vi "TEST-JSON-RPC.vi"() -> ()   [LabVIEW 2019]
uses:
  TEST-JSON-RPC--Cluster.ctl
  <vilib>/JDP Science/JSONtext/JSON Value Type.ctl
  JSON-RPC/JSON-RPC.lvclass/JSON-RPC.ctl
  <vilib>/numeric/Random Number (Range) DBL.vi
  1676b8f3-5053-426b-a1fc-41622b99c0bd.vi
  91eee69d-f7a9-4e42-a9d1-dd5bf5c27f07.vi
  9d079c85-1838-48ae-a1c4-15f57872b121.vi
  423c0946-e876-4033-917c-c4e0f5a656b4.vi
  0ae8443b-0c4b-4e01-b233-50273e00e751.vi
  6f47a901-0ffd-4612-bb45-9ae4cf78a1c3.vi
  f8f63b4b-b52f-497a-b775-281fe5a76cc4.vi
  9d79f0c2-35ce-467d-8164-7d449b6aa026.vi
  53d3177d-6787-4563-b3f2-ec7d47ca270a.vi
  d9266a12-4538-4804-ad7c-12d0542650b7.vi
  JSON-RPC/private/Write ids.vi
  JSON-RPC/private/Read ids.vi
  JSON-RPC/private/Parse Response-JSONtext.vi
  <vilib>/JDP Science/JSONtext/JSON text to Variant (path).vi
  JSON-RPC/private/Parse Response-JSONtext.vi/7ce7fba8-9f44-478d-b6cb-b571ff29f2f5.vi
  JSON-RPC/private/Parse Response-JSONtext.vi/8c905beb-ab4c-49e3-b5c6-2c663b7b30d7.vi
  JSON-RPC/private/Parse Response-JSONtext.vi/fce5892e-0c40-47e1-88e0-6c122aadefe2.vi
  <vilib>/JDP Science/JSONtext/Find Item.vi
  <vilib>/JDP Science/JSONtext/String Subset.vi
  JSON-RPC/private/Create Request-JSONtext.vi
  <vilib>/JDP Science/JSONtext/support/Format JSON Array Text.vi
  <vilib>/JDP Science/JSONtext/JSON text to Variant.vi
  JSON-RPC/private/Create Response-JSONtext.vi
  <vilib>/JDP Science/JSONtext/Get Array Elements.vi
  <vilib>/JDP Science/JSONtext/Get all Object Items.vi
  <vilib>/JDP Science/JSONtext/Parsing/Parse Full Path or Item Name.vi
  <vilib>/JDP Science/JSONtext/Next JSON Value.vi
  <vilib>/JDP Science/JSONtext/support/Error Cluster From Code.vi
  <vilib>/JDP Science/JSONtext/Offset/Find Item Locations by Path.vi
  <vilib>/Utility/error.llb/Error Cluster From Error Code.vi
  <vilib>/Utility/Data Type/Get Type Information.vi
  JSON-RPC/JSON-RPC.lvclass
  <vilib>/JDP Science/JSONtext/LVClass Serializer/JSONtext LVClass Serializer.lvclass
  <vilib>/JDP Science/JSONtext/JSONtext.lvlib
  <vilib>/numeric/Random Number (Range) I64.vi
panel:
  out "Array":T1[](array[typedef])
  out "Names 3":string[](array[string])
  out "Params 3":string[](array[string])
  out "Clusters Section":dbl[](array[numeric])
  out "Arrays":dbl[][](array[numeric])
  out "Clusters":T2[](array[typedef])
  out "Params 2":string[](array[string])
  out "Names 2":string[](array[string])
  out "Params":string[](array[string])
  out "Names":string[](array[string])
  out "REQ.Methods":string[](array[string])
  out "Match?":bool[](array[boolean])
  out "{JSON} Response":string
  out "{JSON} Requests":string
  out "4. parse response":dbl format="%#_6p"
  out "3. create response":dbl format="%#_6p"
  out "2. parse request":dbl format="%#_6p"
  out "1. create request":dbl format="%#_6p"
  out "REQ.Params":string[](array[string])
  out "results":string[](array[string])
  in  "Numeric":i32=3
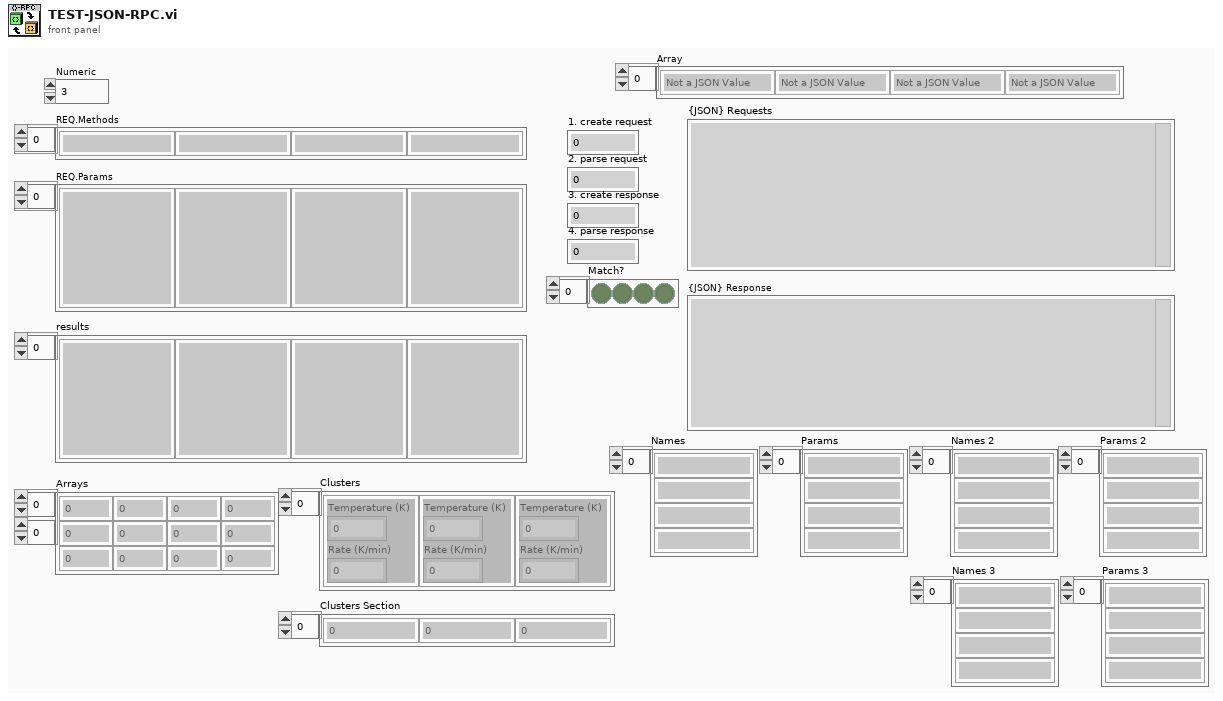
[diagram p1: front panel]
types:
  T1 = typedef "JSONtext.lvlib/JSON Value Type.ctl" = enum16{"Not a JSON Value", "JSON Object", "JSON Array", "String", "Number", "true", "false", "null"}
  T2 = typedef "TEST-JSON-RPC--Cluster.ctl" = cluster{"Temperature (K)":dbl, "Rate (K/min)":dbl}
  T3 = enum16{"Parse Error", "Invalid Request", "Method not found", "Invalid params", "Internal error", "Server error"}
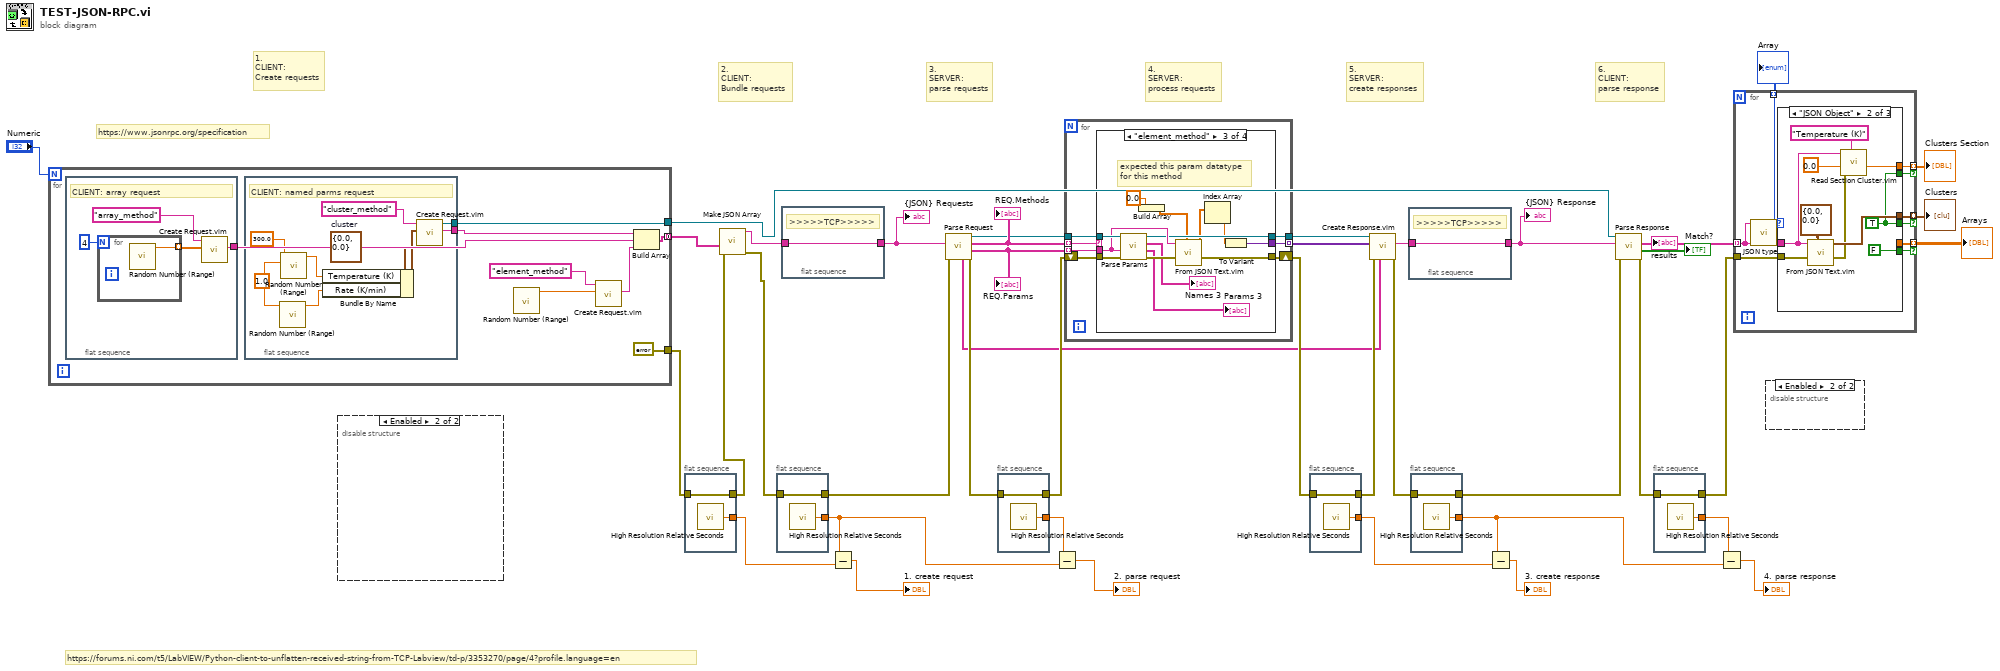
[diagram p0: block diagram]
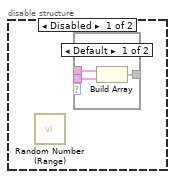
[diagram p2: hidden frame]
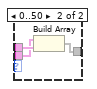
[diagram p3: hidden frame]
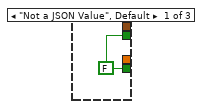
[diagram p5: hidden frame]
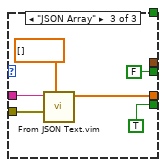
[diagram p6: hidden frame]
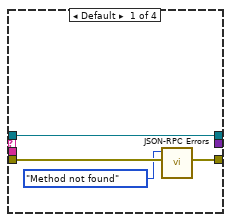
[diagram p7: hidden frame]
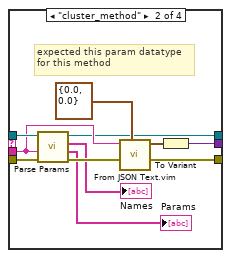
[diagram p8: hidden frame]
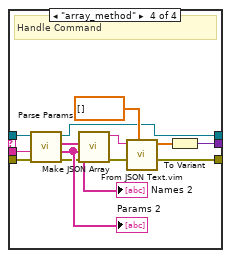
[diagram p9: hidden frame]
diagram:
  # "1.\nCLIENT:\nCreate requests"
  # "3.\nSERVER:\nparse requests"
  # "6.\nCLIENT:\nparse response"
  # "4.\nSERVER:\nprocess requests"
  # "5.\nSERVER:\ncreate responses"
  # "https://forums.ni.com/t5/LabVIEW/Python-client-to-unflatten-received-string-from-TCP-Labview/td-p/3353270/page/4?profile.language=en"
  # "2.\nCLIENT:\nBundle requests"
  # "https://www.jsonrpc.org/specification"
  n1 = for {
    N: "Numeric" -> [_]
    tunnel: [errorcluster {"status"=FALSE, "code"=0, "source"=""} ("error out")] -> w14
    tunnel: [w47] -> w6 mode=concatenating
    tunnel: [w45] -> w2
    n2 = flat-sequence {
      tunnel: [w59] -> w48
      frame #0 {
        # "CLIENT: array request"
        n3 = for {
          N: 4 -> [_]
          tunnel: [w63] -> w60 mode=indexing
          n4 = call-poly <vilib>:"Random Number (Range).vi"() -> ("number"=w63:dbl)  [unwired: 11 in]
        }
        n5 = call "Create Request.vim"("params"=w60, "method"="array_method" ("Request.method")) -> ("{JSON} Requests"=w59:string)  [unwired: 6 in, 3 out]
      }
    }
    n6 = flat-sequence {
      tunnel: [w51] -> w46
      tunnel: [w50] -> w45
      frame #0 {
        w56 = 1.0 ("lower bound (0)")
        w58 = T2 {"Temperature (K)"=0.0, "Rate (K/min)"=0.0}  # cluster
        # "CLIENT: named parms request"
        n7 = call-poly <vilib>:"Random Number (Range).vi"("upper bound (100)"=w56) -> ("number"=w55:dbl)  [unwired: 10 in]
        n8 = call-poly <vilib>:"Random Number (Range).vi"("lower bound (0)"=w56, "upper bound (100)"=300.0 ("lower bound (0)")) -> ("number"=w54:dbl)  [unwired: 9 in]
        n9 = Bundle By Name(cluster=w58, "Temperature (K)"=w54, "Rate (K/min)"=w55) -> (w53:T2)
        n10 = call "Create Request.vim"("params"=w53, "method"="cluster_method" ("Request.method")) -> ("{JSON} Requests"=w51:string, "JSON-RPC out"=w50:refnum<class "JSON-RPC.lvclass">)  [unwired: 6 in, 2 out]
      }
    }
    n11 = call-poly <vilib>:"Random Number (Range).vi"() -> ("number"=w43:dbl)  [unwired: 11 in]
    n12 = call "Create Request.vim"("params"=w43, "method"="element_method" ("Request.method")) -> ("{JSON} Requests"=w42:string)  [unwired: 6 in, 3 out]
    n13 = Build Array(w46, w48, w42) -> (w47:string[])
  }
  n14 = disable-structure shown="Enabled" {
    frame Disabled {
      n15 = call-poly <vilib>:"Random Number (Range).vi"() -> ()  [unwired: 11 in, 1 out]
      n16 = case shown="Default" {
        selector: _ -> [_ _]
        tunnel: _ -> [w66 w69]
        tunnel: _ -> [w65 w68]
        tunnel: [w64 w67] -> _
        frame Default {
          n17 = Build Array(w66, w65) -> (w64:void[])
        }
        frame 0..50 {
          n18 = Build Array(w68, w69) -> (w67:void[])
        }
      }
    }
    frame Enabled {
    }
  }
  n19 = flat-sequence {
    tunnel: [w70] -> w4
    tunnel: [w71] -> w40
    tunnel: w14 -> [w70]
    frame #0 {
      n20 = call <vilib>:"High Resolution Relative Seconds.vi"() -> ("relative seconds"=w71:dbl)
    }
  }
  n21 = call <vilib>:"Make JSON Array.vi"("error in (no error)"=w4, "JSON Elements"=w6) -> ("error out"=w3:errorcluster, "<JSON>"=w5:string)  [unwired: 8 in]
  n22 = flat-sequence {
    tunnel: [w72] -> w23
    tunnel: [w73] -> w36
    tunnel: w3 -> [w72]
    frame #0 {
      n23 = call <vilib>:"High Resolution Relative Seconds.vi"() -> ("relative seconds"=w73:dbl)
    }
  }
  n24 = flat-sequence {
    tunnel: w5 -> [w74]
    tunnel: [w74] -> w21
    frame #0 {
      # ">>>>>TCP>>>>>"
    }
  }
  n25 = Subtract(x=w36, y=w40) -> (x-y=→"1. create request":dbl)
  n26 = call "Parse Request.vi"("error in (no error)"=w23, "{JSON} Request"=w21) -> ("error out"=w22:errorcluster, "Params"=w38:string[], "Methods"=w39:string[], "JSON-RPC out"=w25:refnum<class "JSON-RPC.lvclass">, "IDs"=w12:string[])  [unwired: 5 in]
  "REQ.Params" <- w38
  "REQ.Methods" <- w39
  n27 = flat-sequence {
    tunnel: [w75] -> w37
    tunnel: [w76] -> w33
    tunnel: w22 -> [w75]
    frame #0 {
      n28 = call <vilib>:"High Resolution Relative Seconds.vi"() -> ("relative seconds"=w76:dbl)
    }
  }
  n29 = Subtract(x=w33, y=w36) -> (x-y=→"2. parse request":dbl)
  n30 = for {
    tunnel: w38 -> [w82] mode=indexing
    tunnel: w39 -> [w81] mode=indexing
    tunnel: [w79] -> w13 mode=indexing
    shift-right: [w80] -> w34
    shift-left: w37 -> [w83]
    tunnel: w25 -> [w78]
    tunnel: [w77] -> w24
    n31 = case shown="\"element_method\"" w81 {
      tunnel: w83 -> [w87 w93 w108 w122]
      tunnel: [w86 w98 w111 w113] -> w80
      tunnel: [_ w97 w110 w124] -> w79
      tunnel: w82 -> [_ w91 w106 w121]
      tunnel: w78 -> [w84 w92 w107 w123]
      tunnel: [w84 w90 w105 w112] -> w77
      frame Default {
        n32 = call "JSON-RPC Errors.vi"("error in"=w87, "Enum"=T3."Method not found") -> ("error out"=w86:errorcluster)  [unwired: 9 in]
      }
      frame "cluster_method" {
        # "expected this param datatype\nfor this method"
        n33 = call "Parse Params.vi"("error in (no error)"=w93, "{JSON} Params"=w91, "JSON-RPC in"=w92) -> ("error out"=w94:errorcluster, "Params"=→"Params":string[], "Names"=→"Names":string[], "JSON-RPC out"=w90:refnum<class "JSON-RPC.lvclass">)  [unwired: 5 in]
        n34 = call "From JSON Text.vim"("Data Type and Default Value"=T2 {"Temperature (K)"=0.0, "Rate (K/min)"=0.0} ("Cluster"), "error in (no error)"=w94, "JSON"=w91) -> ("error out"=w98:errorcluster, "Data out"=w95:T2)  [unwired: 7 in]
        n35 = To Variant(anything=w95) -> (Variant=w97:variant)
      }
      frame "element_method" {
        # "expected this param datatype\nfor this method"
        n36 = call "Parse Params.vi"("error in (no error)"=w108, "{JSON} Params"=w106, "JSON-RPC in"=w107) -> ("error out"=w109:errorcluster, "Params"=→"Params 3":string[], "Names"=→"Names 3":string[], "JSON-RPC out"=w105:refnum<class "JSON-RPC.lvclass">)  [unwired: 5 in]
        n37 = Build Array(0.0) -> (w101:dbl[])
        n38 = call "From JSON Text.vim"("Data Type and Default Value"=w101, "error in (no error)"=w109, "JSON"=w106) -> ("error out"=w111:errorcluster, "Data out"=w100:dbl[])  [unwired: 7 in]
        n39 = Index Array(array=w100) -> (element=w99:dbl)  [unwired: 1 in]
        n40 = To Variant(anything=w99) -> (Variant=w110:variant)
      }
      frame "array_method" {
        # "Handle Command"
        n41 = call "Parse Params.vi"("error in (no error)"=w122, "{JSON} Params"=w121, "JSON-RPC in"=w123) -> ("error out"=w114:errorcluster, "Params"=w116:string[], "Names"=→"Names 2":string[], "JSON-RPC out"=w112:refnum<class "JSON-RPC.lvclass">)  [unwired: 5 in]
        "Params 2" <- w116
        n42 = call <vilib>:"Make JSON Array.vi"("error in (no error)"=w114, "JSON Elements"=w116) -> ("error out"=w115:errorcluster, "<JSON>"=w117:string)  [unwired: 8 in]
        n43 = call "From JSON Text.vim"("Data Type and Default Value"=dbl[] [], "error in (no error)"=w115, "JSON"=w117) -> ("error out"=w113:errorcluster, "Data out"=w119:dbl[])  [unwired: 7 in]
        n44 = To Variant(anything=w119) -> (Variant=w124:variant)
      }
    }
  }
  n45 = flat-sequence {
    tunnel: [w125] -> w16
    tunnel: [w126] -> w31
    tunnel: w34 -> [w125]
    frame #0 {
      n46 = call <vilib>:"High Resolution Relative Seconds.vi"() -> ("relative seconds"=w126:dbl)
    }
  }
  n47 = call "Create Response.vim"("ids"=w12, "error in (no error)"=w16, "results"=w13, "JSON-RPC in"=w24) -> ("error out"=w15:errorcluster, "{JSON} Response"=w20:string)  [unwired: 5 in, 1 out]
  n48 = flat-sequence {
    tunnel: w20 -> [w127]
    tunnel: [w127] -> w17
    frame #0 {
      # ">>>>>TCP>>>>>"
    }
  }
  n49 = flat-sequence {
    tunnel: [w128] -> w19
    tunnel: [w129] -> w29
    tunnel: w15 -> [w128]
    frame #0 {
      n50 = call <vilib>:"High Resolution Relative Seconds.vi"() -> ("relative seconds"=w129:dbl)
    }
  }
  n51 = Subtract(x=w29, y=w31) -> (x-y=→"3. create response":dbl)
  n52 = call "Parse Response.vi"("error in (no error)"=w19, "{JSON} Response"=w17, "JSON-RPC in"=w2) -> ("error out"=w18:errorcluster, "Equal?"=→"Match?":bool[], "results"=w10:string[])  [unwired: 4 in, 2 out]
  "results" <- w10
  n53 = flat-sequence {
    tunnel: [w130] -> w11
    tunnel: [w131] -> w30
    tunnel: w18 -> [w130]
    frame #0 {
      n54 = call <vilib>:"High Resolution Relative Seconds.vi"() -> ("relative seconds"=w131:dbl)
    }
  }
  n55 = Subtract(x=w30, y=w29) -> (x-y=→"4. parse response":dbl)
  n56 = for {
    tunnel: w10 -> [w140] mode=indexing
    tunnel: w11 -> [w139]
    tunnel: [w138] -> w8 mode=indexing if=w137
    tunnel: [w136] -> w9 mode=indexing if=w135
    tunnel: [w134] -> w7 mode=indexing if=w133
    tunnel: [w132] -> w1 mode=indexing
    n57 = call <vilib>:"JSON type.vi"("JSON"=w140) -> ("JSON Value Type"=w132:T1)  [unwired: 9 in, 1 out]
    n58 = case shown="\"JSON Object\"" w132 {
      tunnel: w140 -> [_ w147 w157]
      tunnel: w139 -> [_ w150 w156]
      tunnel: [_ _ w154] -> w138
      tunnel: [w141 FALSE TRUE] -> w137
      tunnel: [_ w149 _] -> w136
      tunnel: [w141 w143 FALSE] -> w135
      tunnel: [_ w144 _] -> w134
      tunnel: [_ w143 _] -> w133
      frame "Not a JSON Value", Default {
        w141 = FALSE
      }
      frame "JSON Object" {
        w143 = TRUE
        n59 = call "From JSON Text.vim"("Data Type and Default Value"=T2 {"Temperature (K)"=0.0, "Rate (K/min)"=0.0} ("Cluster"), "error in (no error)"=w150, "JSON"=w147) -> ("error out"=w142:errorcluster, "Data out"=w149:T2)  [unwired: 7 in]
        n60 = call "Read Section Cluster.vim"("Section (Cluster Name)"="Temperature (K)", "error in (no error)"=w142, "Section Cluster"=0.0, "JSON Sections"=w147) -> ("Cluster set from section"=w144:dbl)  [unwired: 4 in, 2 out]
      }
      frame "JSON Array" {
        n61 = call "From JSON Text.vim"("Data Type and Default Value"=dbl[] [], "error in (no error)"=w156, "JSON"=w157) -> ("Data out"=w154:dbl[])  [unwired: 7 in, 1 out]
      }
    }
  }
  "Clusters" <- w9
  "Arrays" <- w8
  "Clusters Section" <- w7
  "Array" <- w1
  n62 = disable-structure shown="Enabled" {
    frame Disabled {
    }
    frame Enabled {
    }
  }
  "{JSON} Requests" <- w21
  "{JSON} Response" <- w17
